vi "Main_02b_Optimized.vi"() -> ()   [LabVIEW 2024]
panel:
  out "Answer 430":i32
  in  "Puzzle":string="24 25 28 31 28\n41 44 45 48 49 50 50\n5 8 10 13 15 16 17 21\n11 13 16 17 19 26\n79 81 78 79 82 84\n16 19 20 18 20 22 25 22\n84 87 90 92 94 97 96 96\n86 87 88 91 88 91 95\n40 43 41 44 49\n8 10 10 11 13\n91 94 95 95 92\n18 19 20 20 21 23 25 25\n15 17 19 19 23\n35 37 37 39 40 43 50\n2 5 6 10 12\n82 85 87 88 91 93 97 94\n30 32 35 38 42 43 43\n64 66 68 72 76\n73 74 77 80 84 86 91\n64 67 72 73 74 76\n72 73 75 81 82 81\n24 25 32 35 37 38 38\n59 60 62 64 65 70 74\n44 46 47 48 50 52 58 63\n54 52 53 56 57 58\n77 76 77 80 82 81\n48 45 48 49 52 54 54\n74 71 74 76 78 81 85\n20 18 19 21 27\n88 86 88 91 92 89 92\n17 16 14 17 18 15\n95 92 91 93 95 96 96\n7 5 6 9 8 11 14 18\n15 12 9 12 14 16 21\n3 2 2 5 6\n58 55 55 57 58 57\n36 35 36 36 36\n73 72 72 75 79\n80 77 78 78 79 82 87\n20 19 23 25 27 28 31 32\n92 90 91 95 97 96\n86 84 86 90 93 96 98 98\n36 33 34 38 41 45\n82 81 85 88 89 92 99\n70 69 71 77 78 81\n51 49 50 57 60 58\n28 27 30 33 35 40 40\n40 37 38 45 49\n53 52 54 55 56 61 67\n27 27 29 31 34\n82 82 84 86 89 92 89\n91 91 93 96 96\n55 55 58 60 64\n80 80 81 82 83 85 88 95\n84 84 87 84 85\n81 81 80 82 79\n25 25 22 24 24\n71 71 74 76 77 74 78\n86 86 87 86 87 88 93\n41 41 43 43 46\n70 70 70 72 71\n12 12 13 13 14 15 15\n23 23 23 26 28 31 35\n84 84 86 88 88 89 91 98\n4 4 5 7 8 9 13 14\n31 31 35 36 37 36\n19 19 23 26 26\n80 80 84 85 88 90 94\n51 51 53 54 58 60 61 66\n35 35 36 42 43\n9 9 12 15 18 24 21\n2 2 8 11 14 15 15\n25 25 30 33 36 38 39 43\n13 13 18 19 26\n10 14 15 17 19\n35 39 40 43 45 46 48 45\n41 45 47 50 50\n16 20 23 25 28 31 34 38\n10 14 15 18 20 25\n42 46 49 46 48\n25 29 32 31 34 31\n7 11 14 11 14 14\n90 94 92 94 98\n27 31 34 32 35 37 44\n50 54 54 56 59 61 63\n48 52 52 53 50\n84 88 89 90 91 91 91\n48 52 54 54 56 60\n85 89 89 91 98\n9 13 15 17 21 23\n43 47 49 52 53 57 55\n76 80 82 83 86 90 93 93\n5 9 11 15 16 20\n53 57 61 62 65 66 73\n65 69 70 73 76 81 82 83\n15 19 21 27 24\n51 55 57 63 65 65\n15 19 22 25 27 33 37\n1 5 6 7 9 11 16 22\n50 56 58 60 63 65 68 70\n36 42 43 44 41\n36 42 44 47 50 52 54 54\n79 84 87 88 90 92 94 98\n35 42 45 46 47 49 52 58\n74 80 83 80 81 82 84 85\n60 67 69 72 73 71 72 71\n85 92 94 97 96 98 98\n17 22 25 27 25 28 32\n22 28 26 28 31 33 40\n51 57 60 61 61 62 63\n7 13 16 16 19 18\n80 87 87 89 89\n70 76 79 81 84 84 88\n39 45 46 49 49 51 52 58\n38 43 45 48 52 55 57 58\n79 84 86 89 93 94 92\n39 45 48 52 52\n58 63 67 69 70 74\n76 83 86 90 97\n13 18 25 27 29 31\n60 66 69 72 75 80 82 81\n21 26 29 31 33 38 38\n31 37 42 45 46 50\n15 21 23 24 30 32 38\n51 48 45 43 44\n45 43 41 40 38 37 36 36\n66 64 61 60 57 53\n89 86 83 81 76\n36 33 30 33 30 29 28 27\n91 88 91 89 86 85 83 85\n12 10 12 11 11\n31 30 27 30 28 27 23\n35 32 31 34 32 26\n11 10 10 9 6 5 4 3\n44 41 38 38 37 35 34 36\n80 78 76 73 72 71 71 71\n45 43 40 37 37 33\n97 94 91 88 87 86 86 80\n58 56 53 51 47 44\n66 63 62 60 58 56 52 53\n73 72 71 68 65 61 61\n95 92 88 86 82\n19 17 16 12 11 10 5\n80 77 74 71 66 64 62 61\n64 62 59 56 51 52\n47 46 43 42 39 38 33 33\n45 44 41 39 34 30\n95 92 89 87 82 81 80 74\n94 96 94 91 88\n89 91 90 88 89\n40 41 38 36 36\n70 72 70 68 67 63\n22 25 24 21 19 18 13\n41 42 39 40 38 37\n35 36 35 32 31 29 32 35\n31 34 31 34 34\n88 90 89 91 90 88 85 81\n54 57 60 59 56 50\n83 85 82 82 80\n66 68 68 65 62 61 62\n35 36 36 34 32 30 30\n79 80 80 78 76 74 70\n44 45 45 43 37\n37 40 37 33 31\n63 65 63 59 56 55 54 56\n19 22 21 17 15 13 11 11\n94 95 91 90 88 84\n22 23 19 18 16 14 7\n29 32 30 23 22\n64 67 64 58 56 57\n29 30 27 24 18 18\n33 36 34 27 24 22 20 16\n50 52 49 48 46 39 37 31\n31 31 28 25 22 21 19 16\n47 47 44 43 40 37 38\n88 88 85 84 84\n41 41 38 36 32\n73 73 70 69 67 66 60\n80 80 81 80 79 77 76 75\n36 36 34 32 34 35\n59 59 57 60 59 58 56 56\n30 30 27 28 25 23 19\n9 9 7 6 5 8 3\n89 89 87 86 85 85 82\n52 52 49 46 46 47\n60 60 59 59 59\n21 21 19 19 15\n17 17 17 16 13 12 10 4\n33 33 29 28 26 25\n67 67 63 61 58 60\n27 27 25 24 20 20\n78 78 76 74 72 68 64\n62 62 59 55 49\n47 47 44 38 36 33 31\n31 31 28 21 23\n81 81 80 79 78 72 72\n75 75 69 66 62\n97 97 91 89 87 85 78\n35 31 28 27 26 25\n35 31 28 27 25 22 21 23\n37 33 32 31 28 28\n73 69 67 65 62 59 55\n67 63 60 58 53\n52 48 47 44 47 46 43\n73 69 70 68 69\n18 14 13 16 16\n91 87 84 81 82 79 77 73\n96 92 90 92 91 88 81\n40 36 35 35 34 33 31\n93 89 86 83 82 82 80 81\n86 82 79 79 78 77 77\n20 16 13 13 12 8\n30 26 23 23 21 19 17 10\n76 72 69 66 62 60 57 54\n57 53 49 46 48\n64 60 58 54 54\n20 16 15 12 8 5 1\n40 36 34 31 27 25 19\n25 21 20 18 16 14 9 6\n48 44 43 40 38 36 29 31\n96 92 90 89 83 81 80 80\n45 41 34 32 28\n35 31 28 27 21 19 14\n35 30 27 26 23\n73 66 63 61 64\n60 55 53 51 50 50\n68 62 61 60 56\n55 50 49 46 43 42 37\n29 23 22 25 22 20 18 16\n96 90 88 85 84 86 83 85\n47 41 39 36 37 37\n72 66 69 68 66 62\n52 47 49 46 43 36\n77 71 68 68 67 66\n99 94 94 93 96\n45 38 35 33 31 31 31\n23 16 13 10 10 6\n33 26 25 25 23 20 18 11\n44 37 33 30 28 27\n90 85 81 79 80\n91 85 82 79 77 73 70 70\n98 91 88 86 82 78\n68 63 61 58 54 52 45\n64 58 57 50 49\n66 59 56 49 52\n89 82 77 76 73 70 70\n80 73 72 67 63\n73 66 60 59 57 50\n11 14 15 17 20 23 21\n47 50 52 55 56 56\n16 17 18 19 20 23 27\n82 83 85 88 90 91 94 99\n59 61 59 61 64 67 70 73\n32 33 36 37 38 36 39 38\n86 89 90 91 89 92 94 94\n67 68 71 68 71 73 76 80\n28 30 31 33 34 32 39\n3 4 6 6 7 10 12 13\n61 64 64 66 69 71 68\n49 50 52 52 53 55 55\n8 11 14 16 16 20\n59 62 62 63 70\n43 45 49 52 55 57\n80 82 86 88 89 92 93 91\n81 82 86 87 88 91 94 94\n38 41 45 48 51 53 57\n35 38 40 41 45 47 54\n6 9 12 14 15 17 22 23\n81 82 83 85 91 90\n74 76 83 84 87 87\n24 27 28 35 37 41\n69 71 72 77 80 85\n12 9 12 13 15 17 20 23\n77 75 76 77 78 81 78\n60 57 59 61 61\n13 10 11 14 16 20\n81 80 81 84 85 90\n6 5 6 7 5 7 10 13\n54 51 54 52 54 55 54\n72 71 70 73 73\n89 86 88 90 91 88 90 94\n8 6 3 5 10\n10 7 8 10 12 12 15 16\n14 11 12 14 16 16 19 18\n39 37 38 38 39 42 44 44\n13 11 12 13 15 15 16 20\n10 8 8 11 14 20\n42 40 42 45 49 50\n67 66 70 73 76 78 77\n32 30 34 35 37 37\n47 44 45 49 51 55\n36 35 39 40 43 45 47 53\n68 66 67 68 73 74\n40 37 38 39 40 46 47 45\n28 26 27 30 35 35\n45 42 48 50 54\n44 43 45 48 54 59\n61 61 62 63 64 66 67\n57 57 58 61 59\n66 66 69 71 73 75 78 78\n59 59 61 64 67 71\n28 28 29 30 31 33 36 41\n41 41 42 41 44 45\n11 11 10 13 15 12\n37 37 40 38 41 41\n41 41 40 42 46\n68 68 69 72 69 71 78\n95 95 95 97 98 99\n9 9 9 10 13 14 17 16\n81 81 82 85 88 88 88\n86 86 86 89 92 96\n58 58 59 62 62 67\n80 80 81 85 87\n84 84 87 91 88\n3 3 7 10 11 12 12\n74 74 75 79 81 82 85 89\n26 26 28 29 31 35 37 44\n38 38 39 46 49\n77 77 80 81 87 88 85\n75 75 78 81 87 90 92 92\n28 28 31 37 40 43 47\n11 11 12 18 20 27\n15 19 21 22 23 26\n58 62 64 65 66 69 71 69\n56 60 61 63 63\n46 50 53 56 58 62\n67 71 73 76 81\n52 56 58 56 58 60\n6 10 11 8 7\n81 85 86 89 87 88 88\n72 76 79 76 79 82 86\n39 43 44 46 43 49\n38 42 45 45 46\n41 45 48 51 51 48\n79 83 86 86 86\n24 28 29 31 33 33 34 38\n55 59 59 61 62 65 67 74\n73 77 80 82 86 87 90\n45 49 50 53 57 54\n80 84 88 90 92 92\n14 18 20 22 24 28 32\n61 65 69 70 73 76 82\n50 54 57 59 62 63 69 70\n75 79 81 82 83 89 92 89\n45 49 52 59 61 63 63\n38 42 44 45 48 55 57 61\n62 66 69 71 74 80 86\n28 35 37 40 41 43\n25 30 32 33 34 37 35\n14 19 20 21 22 22\n8 14 17 20 23 27\n23 28 29 31 38\n68 74 77 78 76 79 80\n14 21 18 20 22 23 25 22\n18 23 20 22 22\n65 72 71 74 76 80\n8 14 15 17 14 17 20 25\n59 65 68 70 70 73\n59 65 68 68 71 74 71\n34 41 43 43 43\n20 25 25 28 32\n43 48 50 50 53 56 58 64\n38 45 49 52 55 58\n23 30 34 35 33\n4 9 11 14 18 20 21 21\n51 57 61 63 67\n67 74 78 81 82 88\n20 26 29 36 37\n9 14 15 18 20 26 29 28\n73 79 82 87 90 90\n9 16 18 24 28\n8 14 19 22 29\n80 77 75 73 76\n93 90 88 85 84 81 78 78\n25 22 20 18 15 12 11 7\n51 48 47 44 42 40 37 31\n77 74 77 75 73 72\n94 91 92 90 88 89\n28 27 26 24 21 22 20 20\n94 91 88 87 86 89 85\n91 90 87 85 82 80 81 74\n59 56 56 54 52 50\n89 88 88 87 84 82 85\n96 95 93 90 89 86 86 86\n25 22 22 19 15\n39 36 34 34 33 31 24\n53 52 49 47 43 40\n93 92 88 85 87\n82 80 76 75 72 69 66 66\n57 55 52 49 47 43 39\n43 40 36 33 26\n33 30 28 21 18\n72 70 67 66 59 61\n26 23 22 19 14 12 10 10\n25 22 20 18 13 10 9 5\n33 30 27 21 19 16 13 6\n96 98 97 95 93 90 89\n47 48 46 45 47\n10 12 9 8 7 5 3 3\n48 49 48 47 43\n25 28 26 25 22 15\n2 4 1 4 3\n59 62 65 64 65\n24 25 22 19 20 17 17\n53 54 52 54 51 48 46 42\n21 23 21 18 19 18 12\n48 49 46 46 43 41 40\n58 61 59 57 57 59\n84 85 83 80 79 78 78 78\n20 22 22 19 17 15 11\n87 89 87 86 86 81\n97 99 95 94 91\n15 18 16 15 11 13\n54 55 53 49 49\n28 30 26 25 23 21 17\n34 37 34 32 28 21\n33 36 33 31 28 21 18 15\n66 69 68 63 61 58 55 58\n93 94 93 87 85 85\n17 18 13 12 8\n81 83 80 78 71 68 63\n68 68 66 65 63\n65 65 62 61 58 57 60\n28 28 26 23 23\n48 48 46 45 44 43 39\n16 16 13 11 6\n30 30 29 26 29 28\n23 23 20 22 20 17 20\n41 41 43 41 41\n39 39 36 39 36 32\n34 34 36 35 30\n88 88 87 85 85 84\n6 6 4 3 3 5\n41 41 38 38 38\n14 14 11 8 8 7 5 1\n75 75 72 72 70 64\n59 59 55 52 51\n91 91 88 84 81 79 80\n95 95 92 88 85 85\n62 62 60 59 55 51\n17 17 13 11 4\n67 67 66 65 63 58 56\n63 63 56 55 57\n46 46 45 39 39\n42 42 39 38 32 28\n91 91 86 84 78\n30 26 24 22 21 20 19\n58 54 53 50 53\n10 6 5 4 4\n93 89 88 86 85 83 81 77\n52 48 46 43 38\n89 85 84 81 83 82 79\n46 42 41 39 42 44\n48 44 41 44 43 42 39 39\n61 57 56 53 54 51 47\n55 51 54 52 50 43\n23 19 16 16 15 13 11 8\n23 19 17 16 14 14 13 14\n23 19 19 17 14 11 9 9\n24 20 19 16 14 14 10\n94 90 88 85 85 84 77\n47 43 41 39 36 32 30\n54 50 46 45 42 43\n88 84 81 77 77\n29 25 21 20 18 15 12 8\n67 63 59 58 51\n16 12 6 3 1\n68 64 61 59 53 51 50 53\n70 66 60 58 58\n84 80 75 73 70 66\n92 88 86 85 78 77 71\n93 86 83 82 79 77 74 73\n56 50 48 46 48\n25 20 19 16 13 13\n79 74 73 72 70 69 67 63\n77 71 70 67 64 62 56\n80 74 71 68 67 69 68 65\n36 29 27 26 28 31\n88 82 83 82 82\n13 6 5 7 3\n17 11 12 9 6 1\n87 82 81 80 80 78 75\n23 17 14 11 11 12\n70 64 61 58 58 58\n96 91 90 87 87 85 81\n92 85 85 83 80 74\n23 17 13 12 11\n70 63 59 56 55 53 54\n85 80 79 76 73 70 66 66\n81 75 74 73 72 68 64\n69 62 59 55 54 49\n68 62 60 58 52 49\n81 75 74 71 69 64 66\n71 65 58 55 55\n39 32 31 26 24 22 19 15\n53 47 42 40 33\n39 40 43 44 46 48 55 61\n41 37 35 31 29 25\n33 28 26 23 23 24\n53 49 48 45 43 39\n45 45 46 47 49 49 50 57\n55 52 51 50 47 46 46 42\n43 40 39 33 27\n31 37 42 44 46 46\n38 36 34 33 30 29 27 30\n25 31 33 35 32 38\n74 74 80 82 83 87\n34 40 40 41 44 45 50\n75 68 66 63 61\n72 69 67 64 61 54 54\n23 27 27 29 34\n53 57 58 60 60\n47 40 35 34 35\n28 24 22 20 18 16 16\n55 58 56 52 52\n9 9 11 14 15 12 16\n38 33 29 27 26 21\n19 18 19 19 20 24\n59 59 55 54 53 52 46\n9 13 16 18 20 21 22 26\n36 32 25 24 21 15\n40 41 44 45 47 46 49 53\n2 4 7 7 9 11 18\n16 21 20 22 23 25\n90 84 82 79 75 72 68\n74 74 78 79 81 81\n59 61 64 63 61 59 52\n76 76 75 68 67 64 65\n85 85 85 86 85\n34 37 35 32 29 25 24\n86 84 84 83 80 77 75 68\n15 16 20 21 23 26 29\n65 71 75 76 73\n95 95 94 91 88 90\n81 87 88 91 94 96 97 97\n4 8 11 13 14 12 15\n34 40 42 44 47 45 43\n34 36 38 41 48 51 55\n44 46 44 44 41 40 38 38\n95 98 97 96 93 93\n54 53 50 48 44 38\n25 25 23 20 17 15 11\n82 82 81 81 81\n52 56 58 62 64 68\n39 39 36 35 34\n83 86 88 85 87\n46 39 41 40 34\n18 24 27 34 37\n34 30 28 26 24 23 24\n65 67 70 72 74 77 76\n18 23 24 27 34 36 37 36\n10 10 11 14 16 21\n2 6 9 12 13 13 15 14\n46 51 52 56 57 59 63\n69 75 80 81 85\n60 61 64 61 58 57 60\n84 87 86 80 79 79\n76 73 75 73 73\n72 66 65 62 65 63 60\n10 14 16 17 18 25 27 31\n15 16 17 17 18\n94 94 91 86 82\n39 46 47 49 52 56 58\n1 1 2 2 2\n3 7 8 10 17 20 20\n26 26 24 19 17 14 12\n43 43 42 44 42 37\n62 62 59 60 59 58 55 55\n19 23 27 28 30 36\n41 44 42 44 41 41\n12 10 10 12 13 15 17 22\n52 53 54 55 62 65 67 67\n21 22 21 20 20 19 16 17\n50 46 45 43 41 40 40 40\n69 70 74 77 77\n83 87 89 89 90 94\n14 11 9 11 15\n86 83 84 88 89 92 93 97\n47 44 44 47 47\n83 87 89 89 92\n65 61 57 55 57\n65 69 71 75 78 81 81\n72 72 73 80 81 84 82\n31 28 30 34 35 36 39 41\n94 89 83 82 81 80 79\n55 55 52 48 45 45\n64 66 64 61 59 54 50\n7 6 11 14 17 21\n83 79 75 73 72 71 70 70\n37 36 36 33 31 29 28 31\n92 94 93 92 91 86\n71 70 69 68 63\n80 83 82 83 82 79 77\n51 55 57 61 58\n53 50 47 46 42 42\n89 89 90 96 99\n34 33 36 39 40 44 42\n77 73 69 68 66\n10 10 13 14 16 13\n76 77 74 74 69\n91 92 93 95 96 99 99 99\n17 15 11 10 9 6 5\n47 47 44 41 39 40 41\n21 25 28 30 28 35\n52 55 52 48 49\n44 44 42 45 43 39\n36 36 37 41 42 44 46 44\n43 43 40 40 37 40\n19 22 19 15 10\n61 62 59 56 55 51\n31 37 38 41 45 45\n1 5 8 9 10 15\n42 38 40 38 37 30\n60 61 59 57 55\n36 34 36 33 30\n38 40 41 42 40 42 44 43\n58 55 53 52 51 49 46 42\n91 88 91 89 88 89\n53 53 51 50 50\n89 91 92 95 92 99\n18 13 15 13 11 11\n64 65 66 68 69 70\n71 74 77 80 83 84 86\n40 42 45 48 51 52 54 57\n29 31 32 34 37 39 42\n13 14 15 18 19 22 25 27\n20 18 16 13 12\n21 19 16 13 12 10 7\n88 91 94 95 97\n25 22 21 18 15 13\n55 53 51 48 45 42 40 38\n63 62 61 58 55 52 50 48\n61 58 56 55 54 52 49\n59 60 62 65 67 69\n68 69 72 74 76 77\n73 70 68 65 63 61\n88 89 92 95 96\n37 36 34 33 30\n50 51 52 55 56 59 62 63\n67 70 71 73 76 78\n90 92 93 95 96\n41 42 43 45 46\n60 59 56 54 52 50 47\n39 38 36 35 32 31 28 27\n14 17 19 20 21 24 25\n60 58 56 55 53 51\n11 10 7 6 5\n10 11 14 15 17 19\n14 11 8 5 4 3\n64 62 61 58 55 52 51\n17 14 13 12 11 10 7\n72 70 69 68 66 64 61\n74 77 80 82 85 86 88 89\n26 29 32 35 36 38\n62 60 59 57 56 53 50\n26 25 23 22 20 19 16 13\n7 10 13 16 17 20 21\n71 70 69 67 65 62 61\n11 13 14 15 18 21\n22 20 17 14 11 9 6 5\n3 4 6 8 11 12 14 15\n2 4 6 9 12\n81 84 86 88 91 94 97 98\n32 33 36 37 38 41\n78 77 76 74 73\n71 72 74 76 78\n44 45 48 49 51 53 54\n78 75 74 73 70 69 66 64\n75 74 71 69 66 63\n84 82 79 78 75 74 71 69\n62 61 58 56 54 52 51 48\n98 95 92 89 88 87 85\n3 5 7 9 10 12 14\n89 87 85 83 82\n80 79 77 75 73 71 68\n61 62 64 66 69 72 74 76\n51 49 46 44 43 40 39 38\n70 67 64 63 62\n35 34 33 31 29 27 24 23\n42 44 47 50 51 52\n52 55 58 59 62 64 65\n67 69 72 74 77 80\n14 12 11 9 8\n53 51 48 45 43\n57 58 60 63 65 68 70\n30 32 35 36 38 41 43\n99 97 96 94 91 89 88\n68 65 63 61 59 57 56\n92 90 88 86 85\n44 46 47 49 52\n49 52 53 54 56 57 59\n28 27 25 22 21 20 17 16\n48 46 43 41 40\n79 80 82 85 87 88 89\n58 56 54 53 52 51 49 47\n54 57 60 61 62 64 65\n40 39 38 36 35 33\n32 30 29 27 24 23 22\n17 14 11 9 7 5\n91 89 88 87 86 83\n19 16 14 11 9 8\n40 41 42 45 46 49 51 52\n86 84 81 80 77 74 71 68\n42 41 39 37 36 34\n36 33 32 29 26 23 20\n24 21 20 17 16\n12 9 8 5 4\n76 79 82 85 88 91 92\n64 66 69 72 75\n35 37 38 41 44 46 49 51\n94 92 89 87 86 85\n66 68 71 74 76\n81 80 79 77 75 74 72 71\n83 86 89 92 94\n43 40 37 34 31\n36 37 38 41 43\n31 28 25 23 20 18\n45 44 42 41 38 36\n86 85 84 82 80 77 74\n58 57 55 54 53 50 49 47\n70 71 73 75 78\n73 76 79 80 82\n85 83 81 78 75 72\n37 38 39 42 45 48 50\n64 67 68 71 72\n66 63 61 58 56\n61 64 65 67 68 69 72 74\n95 94 91 90 89 87 85 84\n84 87 89 91 94\n63 65 68 71 72 73\n40 39 38 37 35 34 32\n88 87 86 83 82 81 80\n71 70 68 65 63 62\n92 90 88 85 82 81 80\n76 74 71 68 65 64\n9 11 12 14 17\n74 75 77 78 80 82\n30 33 36 38 39 42 44 45\n59 62 63 65 67 69\n83 86 88 91 94 95\n29 28 26 23 21\n70 71 74 77 78 80 82\n70 72 74 75 76\n6 9 12 15 18 21 24 25\n32 31 29 26 23 22\n76 75 74 72 70 68\n93 92 91 90 89\n56 58 59 60 63 64\n72 73 74 76 78 80 83 85\n96 95 92 89 86 84\n98 95 94 93 90\n27 29 31 33 36 37 39 40\n48 47 44 41 39 38 37 36\n20 19 16 14 13\n98 97 96 95 92\n71 72 74 75 78 80\n49 51 53 55 57\n63 60 59 56 53\n78 80 82 83 84\n80 79 77 75 73 71 69 66\n24 25 27 30 33 34 36\n81 82 84 86 89\n35 36 39 42 43 44 46\n14 15 16 18 21 23 25 28\n83 84 86 89 92 93\n82 81 78 76 73\n19 21 24 27 28 30 32\n61 60 58 56 53\n7 8 10 12 14\n69 67 66 64 61 59\n29 28 25 23 21\n44 46 49 52 54 55 57 60\n6 7 9 10 12 14 15\n27 25 22 19 18 17 14\n50 52 54 56 59 60 63 65\n40 39 36 33 32\n10 11 12 14 16\n30 27 26 24 23 21 19 18\n24 22 20 19 18 16 14\n89 91 93 95 97 98 99\n60 57 54 53 51 48 47\n1 3 6 7 8 10 13\n14 13 11 10 8\n57 55 53 51 50\n48 46 45 42 40 39 36 35\n42 43 45 47 50\n92 90 88 86 85 82\n94 91 90 88 87 85 84 82\n45 46 48 50 53\n24 21 20 17 14 11 9 7\n65 64 62 60 59 56 55 53\n54 51 50 48 47 44 43\n49 47 45 42 39 38 37 34\n37 34 32 30 27 26 25\n87 88 91 92 94 97\n86 84 81 79 76 73 71 70\n59 60 63 64 65\n39 42 43 44 46\n14 16 17 18 21 23 24 27\n5 6 7 9 12 14 16 19\n64 65 67 70 73\n90 89 88 85 84 81 78\n83 85 88 90 92 93 96 97\n83 81 79 76 74 73\n68 71 74 77 78 80 83 86\n41 40 38 35 34\n34 31 28 27 24\n87 88 90 92 93 94 96\n52 55 56 57 60 62\n17 20 23 24 25 27\n30 28 27 24 21 18 15 12\n28 27 26 25 22 19\n72 69 68 67 66 64\n59 56 55 54 52 49 47 45\n26 28 31 32 35 36 38\n52 49 46 45 42 41 39\n9 10 11 12 14 15 17\n35 36 37 39 40 42 44 47\n59 58 55 54 53 52\n11 10 9 8 6 4 3\n18 20 22 23 24 27\n10 8 7 6 5 4 3\n68 71 72 74 76 77\n64 63 62 59 56 54 51\n37 36 35 33 31 28\n98 97 96 95 93 92 90 87\n18 19 21 24 27\n23 24 26 29 30 33 36 39\n52 51 49 47 46 45 42 41\n50 48 47 44 43\n40 43 46 49 52 54 55 58\n45 43 40 37 35 33 31 29\n35 33 30 27 24 23 20 18\n82 83 84 86 88\n19 16 13 10 9\n37 34 33 32 29\n86 83 80 77 76\n77 78 79 81 84 87 88 90\n13 15 18 21 22 25 27\n6 7 9 11 13 14 17 18\n51 50 48 47 46 44 41 40\n79 80 82 83 85\n74 72 69 67 65 63 62 59\n58 57 55 53 50\n54 57 60 62 64 65 68\n28 30 32 34 37 38\n10 13 15 18 20 22 24 27\n80 79 77 74 73 71 70\n21 20 18 15 13 11 9\n21 23 26 29 31 33 35\n74 75 76 78 81 83\n61 58 56 55 54 53 51 50\n54 55 56 57 60 62 64 65\n45 43 42 41 38 37 35 34\n47 50 53 56 57 59\n98 95 94 93 92 90\n13 12 9 7 6 4 2\n68 70 73 76 79 80 81 84\n59 62 65 68 69 72 75\n80 82 84 87 89 92 95\n63 65 68 70 71 72 73 76\n92 90 87 86 85 82 80 77\n20 18 15 13 11 9 7\n60 59 58 55 54 51 48 47\n18 16 15 13 11 9\n71 68 65 62 61 59 57\n69 68 65 62 60 57 56\n75 74 73 72 70 67 65 62\n17 20 22 25 28 31\n43 45 46 48 50 51\n28 25 22 21 19 17 15\n36 33 30 29 27 24 22 21\n13 14 15 18 20 23\n84 82 81 78 77 76 75\n23 26 27 30 33\n56 53 50 47 46\n25 27 28 30 31 32 34 37\n90 92 94 95 96 99\n82 83 85 88 90 92 95\n49 46 45 43 42 40\n55 58 61 63 65 68 69 72\n61 62 65 66 68 69\n49 52 54 55 56 58 59 61\n41 43 44 46 49\n74 71 70 68 65 62 61 58\n26 29 30 31 32 35 38 40\n11 12 14 15 18 21\n79 76 74 72 71 68 66\n17 20 23 25 27 30 33 35\n52 53 55 58 60\n6 7 9 11 12\n88 85 84 83 81 79 77\n71 74 76 77 79\n70 72 75 78 79\n54 56 58 59 62\n97 96 94 91 90\n6 9 10 11 14 17 20 22\n23 21 18 15 14\n99 98 96 94 91 88 87\n96 93 92 90 89 88\n91 89 88 85 84 82 80 77\n86 87 88 91 94\n3 4 7 10 11 12\n56 59 61 64 67\n40 41 44 46 48 49 52 53\n35 34 32 31 30 27 24 22\n48 47 44 43 42 40 38 36\n31 29 26 23 20 19 16\n25 27 28 29 30 32\n4 7 10 13 15\n36 39 40 42 43 45 48\n20 23 25 27 28 31 34\n40 42 45 48 49 52 54\n14 12 10 9 7 4 2 1\n76 74 71 68 66 64\n25 27 29 30 31\n34 31 29 28 25 24 22\n63 64 67 70 72 73\n95 93 90 89 87 85\n29 27 25 22 20 18\n28 30 32 33 34 37\n53 52 49 46 43 42\n41 40 38 36 33 31 30\n81 79 77 75 74 73\n97 96 95 94 93 90\n77 79 81 82 83\n67 64 62 59 56 54\n55 54 52 50 48 46 45\n74 73 70 69 67\n90 88 85 82 80\n16 14 13 12 11\n32 31 29 26 24 23\n17 18 21 24 27\n21 18 16 14 11 9 6\n37 39 41 42 45 47\n6 8 9 11 13\n35 34 32 30 28 27 25 23\n80 78 77 75 73 71\n4 5 6 9 12 15\n48 51 52 53 55 56 57\n31 33 34 35 37 38 40 42\n75 77 78 80 83 86 87\n39 40 43 46 49 51\n70 71 72 74 75 77 79\n95 92 89 87 85 84 82\n5 7 10 12 14 17 18 20\n68 67 66 65 62\n61 63 64 66 68 69 70 73\n61 59 57 55 53 51\n38 36 33 32 31 30 29\n83 82 79 76 75 74 72 69\n17 20 22 23 26 28\n81 83 86 87 90 93 94\n85 82 81 79 77\n7 10 11 12 13\n94 93 90 87 84 82\n63 64 66 69 70 71 73\n35 36 37 39 42 45\n48 47 45 44 41\n93 92 91 89 88 86\n47 50 52 54 55\n33 35 38 40 43 46 48 49\n70 73 76 77 80\n96 95 92 91 88 87 84 83\n14 17 20 21 22 23 25 28\n14 15 16 17 18 20 21\n72 71 70 68 65 63 60 59\n57 60 61 64 67 68\n18 17 16 13 10\n49 47 44 42 40 38\n30 32 34 37 38\n70 69 68 65 63 62 61\n37 40 43 44 47 48\n55 54 53 52 50 47 45\n90 88 86 85 83 81 80\n90 88 85 83 80\n38 40 43 45 46\n64 67 70 73 75\n91 93 95 98 99\n18 15 12 9 8 6 4 1\n80 77 75 73 70 67 64 62\n29 26 24 21 19 16 15\n61 63 64 67 69 72\n60 59 57 54 53\n63 61 59 57 56 54 53\n49 50 52 53 54\n57 59 60 63 66\n61 63 64 65 66 67 69 70\n24 21 19 18 16 14\n42 39 36 35 34 33\n95 94 92 91 89 86 83\n72 75 77 78 81 83 86\n4 5 6 8 9 12 14\n20 22 25 28 30 33\n65 68 70 71 73 74\n1 3 4 6 9 11 12 15\n75 77 79 81 83 85\n21 22 25 28 29 31 34\n8 7 4 3 2\n39 37 34 31 28"
  in  "Example":string="7 6 4 2 1\n1 2 7 8 9\n9 7 6 2 1\n1 3 2 4 5\n8 6 4 4 1\n1 3 6 7 9"
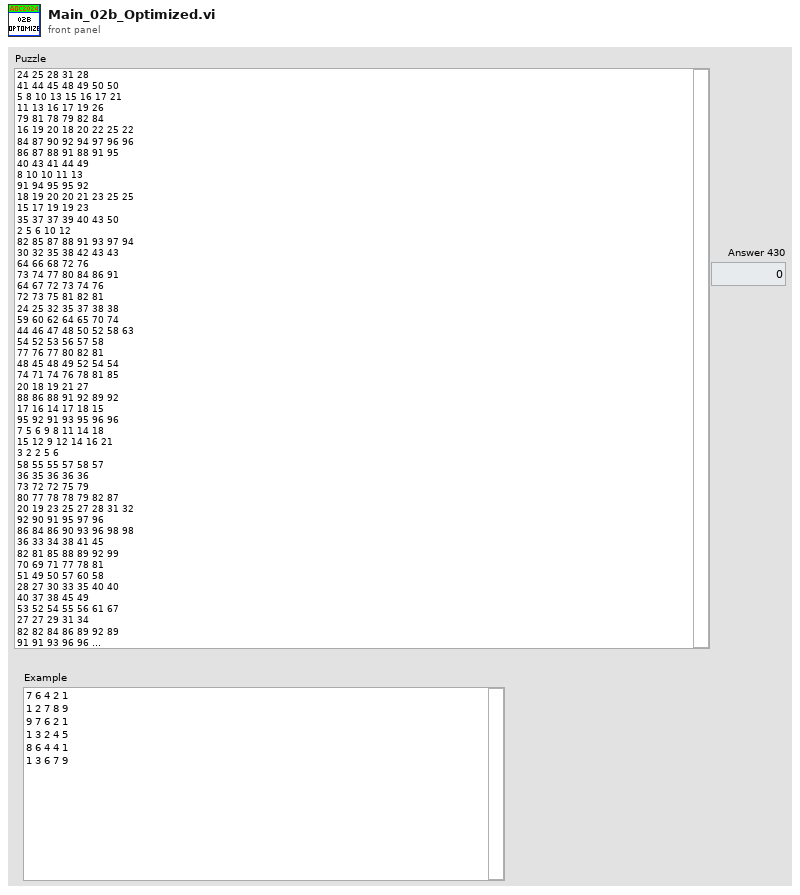
[diagram p1: front panel]
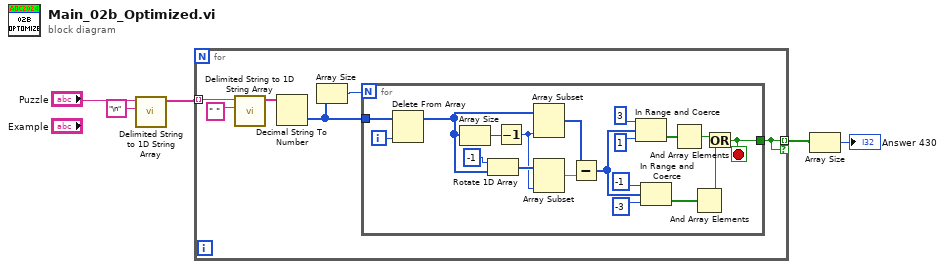
[diagram p0: block diagram]
diagram:
  n1 = call <vilib>:"Delimited String to 1D String Array.vi"("delimiter"="\n", "delimited string"="Puzzle") -> ("string array"=w1:string[])  [unwired: 9 in]
  n2 = for {
    tunnel: [w6] -> w5 mode=indexing if=w6
    tunnel: w1 -> [w8] mode=indexing
    n3 = call <vilib>:"Delimited String to 1D String Array.vi"("delimiter"=" ", "delimited string"=w8) -> ("string array"=w9:string[])  [unwired: 9 in]
    n4 = Decimal String To Number(string=w9) -> (number=w7:i32[])  [unwired: 2 in, 1 out]
    n5 = Array Size(array=w7) -> (size(s)=w11:i32)
    n6 = for {
      N: w11 -> [_]
      tunnel: w7 -> [w13]
      tunnel: [w19] -> w6
      i -> [w12]
      stop <- w19 stop-if-true
      n7 = Delete From Array(array=w13, index=w12) -> (array with subset deleted=w14:i32[])  [unwired: 1 in, 1 out]
      n8 = Array Size(array=w14) -> (size(s)=w28:i32)
      n9 = Rotate 1D Array(1:w14, 2:-1 ("n")) -> (0:w29:i32[])
      n10 = Decrement(x=w28) -> (x-1=w27:i32)
      n11 = Array Subset(array=w14, length=w27) -> (w26:i32[])  [unwired: 1 in]
      n12 = Array Subset(array=w29, length=w27) -> (w25:i32[])  [unwired: 1 in]
      n13 = Subtract(x=w26, y=w25) -> (x-y=w20:i32[])
      n14 = In Range and Coerce(upper limit=3, x=w20, lower limit=1) -> (In Range?=w17:bool[])  [unwired: 1 out]
      n15 = In Range and Coerce(upper limit=-1, x=w20, lower limit=-3) -> (In Range?=w18:bool[])  [unwired: 1 out]
      n16 = And Array Elements(Boolean array=w17) -> (logical AND=w16:bool)
      n17 = And Array Elements(Boolean array=w18) -> (logical AND=w15:bool)
      n18 = Or(x=w16, y=w15) -> (x .or. y?=w19:bool)
    }
  }
  n19 = Array Size(array=w5) -> (size(s)=→"Answer 430":i32)
